vi "Check Action.vi"(6 "HRS Time":dbl, 7 "Values In":dbl[](array[numeric]), 8 "error in (no error)":errorcluster, 11 "SequencedValves in":refnum<class "SeqDelayControl.lvclass">) -> (0 "error out":errorcluster, 1 "Do Action":bool, 2 "Action":T1, 3 "SequencedValves out":refnum<class "SeqDelayControl.lvclass">, 5 "Values":dbl[](array[numeric]))   [LabVIEW 2020, in "VolatusControl.lvlib" / "SeqDelayControl.lvclass"]
uses:
  SeqDelayControl.lvclass
  Valve Action.ctl
  Volatus/MessageQ/MessageQ.lvclass
  SeqDelayControl.lvclass/SeqDelayControl.ctl
  State.ctl
  VolatusControl.lvlib
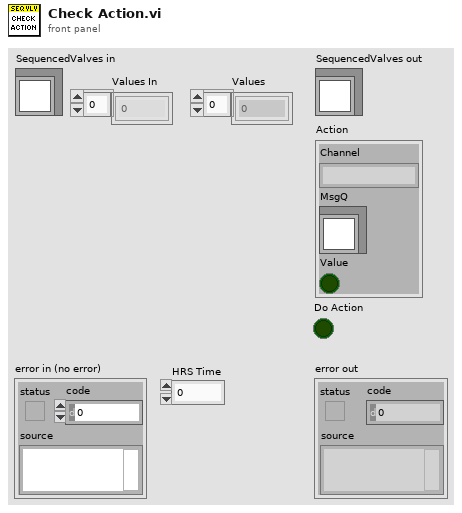
[diagram p1: front panel]
types:
  T1 = typedef "VolatusControl.lvlib/Valve Action.ctl" = cluster{"Channel":string, "MsgQ":refnum<class "MessageQ.lvclass">, "Value":bool}
  T2 = typedef "VolatusControl.lvlib/SeqDelayControl.lvclass/State.ctl" = enum16{"Idle", "Start", "Delay"}
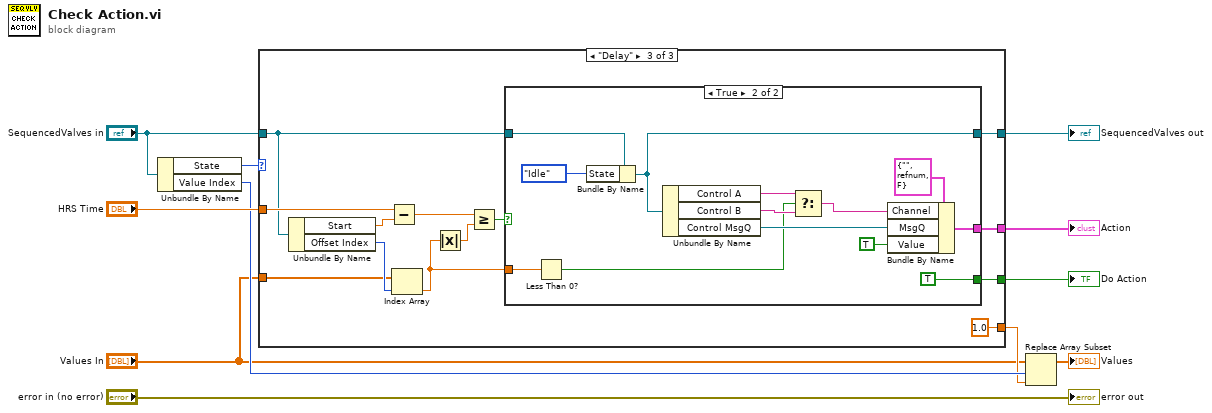
[diagram p0: block diagram]
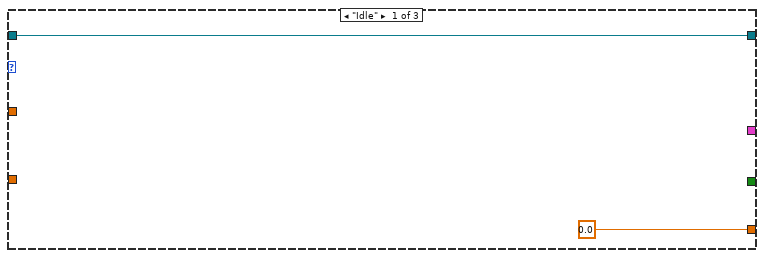
[diagram p2: hidden frame]
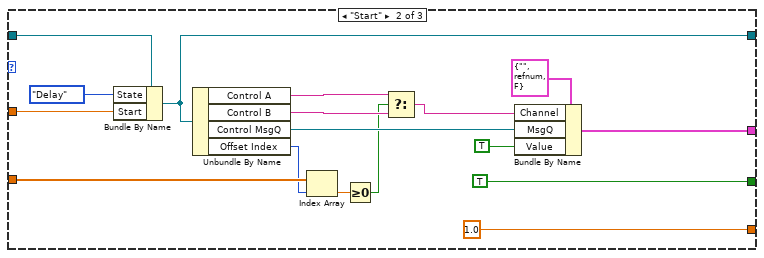
[diagram p3: hidden frame]
diagram:
  n1 = Unbundle By Name("SequencedValves in") -> ("State"=w10:T2, "Value Index"=w3:i32)
  n2 = case shown="\"Delay\"" w10 {
    tunnel: "SequencedValves in" -> [w13 w27 w39]
    tunnel: "HRS Time" -> [_ w25 w43]
    tunnel: [w13 w24 w38] -> w7
    tunnel: [_ w29 w37] -> w6
    tunnel: [_ TRUE w36] -> w5
    tunnel: [0.0 1.0 1.0] -> w2
    tunnel: "Values In" -> [_ w20 w34]
    frame "Idle" {
    }
    frame "Start" {
      n3 = Bundle By Name(cluster=w27, "State"=State."Delay", "Start"=w25) -> (w24:refnum<class "SeqDelayControl.lvclass">)
      n4 = Unbundle By Name(w24) -> ("Control A"=w16:string, "Control B"=w17:string, "Control MsgQ"=w23:refnum<class "MessageQ.lvclass">, "Offset Index"=w19:i32)
      n5 = Index Array(array=w20, index=w19) -> (element=w18:dbl)
      n6 = Greater Or Equal To 0?(x=w18) -> (x >= 0?=w15:bool)
      n7 = Select(t=w16, s=w15, f=w17) -> (s? t:f=w14:string)
      n8 = Bundle By Name(cluster=T1 {"Channel"="", "MsgQ"=refnum, "Value"=FALSE} ("Action"), "Channel"=w14, "MsgQ"=w23, "Value"=TRUE) -> (w29:T1)
    }
    frame "Delay" {
      n9 = Unbundle By Name(w39) -> ("Start"=w42:dbl, "Offset Index"=w35:i32)
      n10 = Subtract(x=w43, y=w42) -> (x-y=w41:dbl)
      n11 = Index Array(array=w34, index=w35) -> (element=w31:dbl)
      n12 = Absolute Value(x=w31) -> (abs(x)=w32:dbl)
      n13 = Greater Or Equal?(x=w41, y=w32) -> (x >= y?=w40:bool)
      n14 = case shown="True" w40 {
        tunnel: w39 -> [w44 w52]
        tunnel: [w44 w51] -> w38
        tunnel: [_ w54] -> w37
        tunnel: [_ TRUE] -> w36
        tunnel: w31 -> [_ w47]
        frame False {
        }
        frame True {
          n15 = Less Than 0?(x=w47) -> (x < 0?=w46:bool)
          n16 = Bundle By Name(cluster=w52, "State"=State."Idle") -> (w51:refnum<class "SeqDelayControl.lvclass">)
          n17 = Unbundle By Name(w51) -> ("Control A"=w49:string, "Control B"=w48:string, "Control MsgQ"=w55:refnum<class "MessageQ.lvclass">)
          n18 = Select(t=w49, s=w46, f=w48) -> (s? t:f=w45:string)
          n19 = Bundle By Name(cluster=T1 {"Channel"="", "MsgQ"=refnum, "Value"=FALSE} ("Action"), "Channel"=w45, "MsgQ"=w55, "Value"=TRUE) -> (w54:T1)
        }
      }
    }
  }
  "SequencedValves out" <- w7
  "Action" <- w6
  "Do Action" <- w5
  n20 = Replace Array Subset(array="Values In", new element=w2, index=w3) -> (→"Values":dbl[])
  "error out" <- "error in (no error)"
